vi "PR4000 init.vi"(3 "VISA Refnum in":refnum<visa-resource-name>) -> (0 "error out":errorcluster, 1 "VISA Refnum out":refnum<visa-resource-name>)   [LabVIEW 2023]
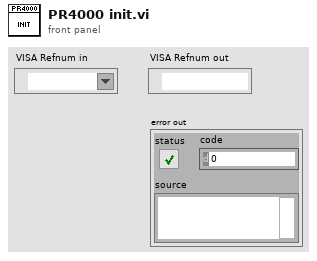
[diagram p1: front panel]
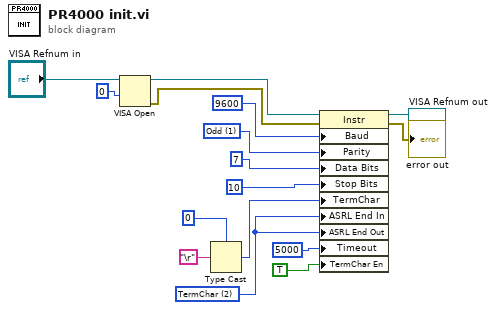
[diagram p0: block diagram]
diagram:
  w13 = u16 1 items=["None", "Odd", "Even", "Mark", "Space"] ("Serial Settings:Parity (Odd)")
  w8 = u16 2 items=["None", "Last Bit", "TermChar"] ("Serial Settings:End Mode for Reads")
  n1 = VISA Open(access mode=u32 0, VISA resource name="VISA Refnum in") -> (VISA resource name=w4:refnum<visa-resource-name>, error out=w5:errorcluster)  [unwired: 3 in]
  n2 = Type Cast(type=u8 0, x="\r") -> (*(type *) &x=w7:u8)
  n3 = property class="Instr"(reference=w4, error in=w5, "Baud"=u32 9600 ("Serial Settings:Baud Rate"), "Parity"=w13, "Data Bits"=u16 7 ("Serial Settings:Data Bits (7)"), "Stop Bits"=u16 10 ("ASRL Stop Bits"), "TermChar"=w7, "ASRL End In"=w8, "ASRL End Out"=w8, "Timeout"=u32 5000 ("General Settings:Timeout Value"), "TermChar En"=TRUE ("Message Based Settings:Termination Character Enable")) -> (reference out=→"VISA Refnum out":refnum<visa-resource-name>, error out=→"error out":errorcluster)
